vi "main.vi"() -> ()   [LabVIEW 2016]
uses:
  global/Config_Infos.vi
  <vilib>/registry/registry.llb/Registry RtKey.ctl
  <vilib>/registry/registry.llb/Read Registry Value Simple STR.vi
panel:
  out "String/Binary data":string
  in  "config file":path=path "C:/Users/guigue/Documents/hardware/software_config/rga/RGAConfig.ini"
  in  "stop":bool
  in  "Tab Control":enum32{"Status", "Ping listener", "Log"}(tab)
  in  "saving?":bool
  in  "filament?":bool
  out "status display":u16(ring)=5 items=["Filament on/Saving off", "Waiting 1", "Filament on/Saving on", "Waiting 2", "Filament off/Saving off", "Idle"]
  out "Init OK?":bool
  out "error initialization (out)":errorcluster
  out "broadcast.ping listener?":bool=TRUE
  in  "is_running?":bool
  in  "is_stopping?":bool
  out "broadcast.ping error out":errorcluster
  out "Execution:State":T1(ring)
  out "service log":string
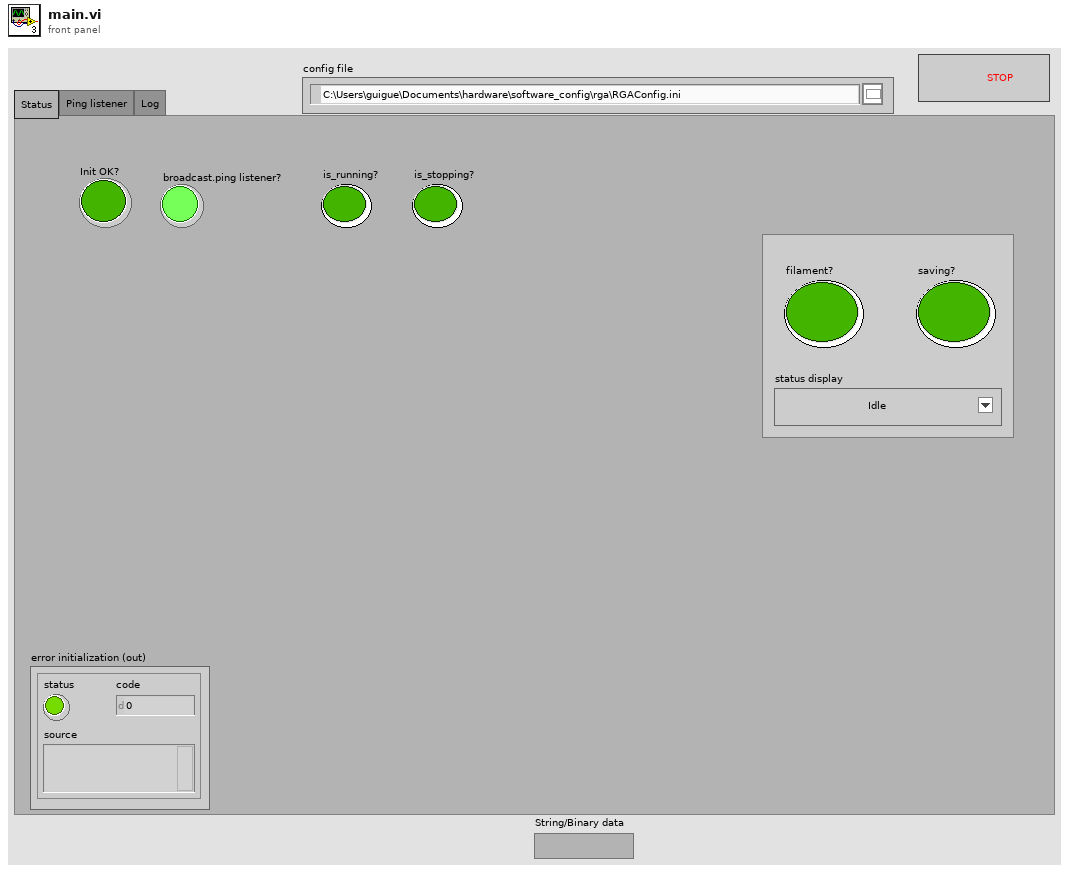
[diagram p1: front panel]
types:
  T1 = enum32{"Bad", "Idle", "Run top level", "Running"}
  T2 = typedef "Registry RtKey.ctl" = enum32{"HKEY_CLASSES_ROOT", "HKEY_CURRENT_USER", "HKEY_LOCAL_MACHINE", "HKEY_USERS", "HKEY_PERFORMANCE_DATA", "HKEY_CURRENT_CONFIG", "HKEY_DYN_DATA"}
  T3 = typedef "Registry refnum.ctl" = refnum<k1>
  T4 = cluster{"stop":refnum<vi>, "is_running?":refnum<vi>, "is_stopping?":refnum<vi>, "filament?":refnum<vi>, "saving?":refnum<vi>, "status display":refnum<vi>}
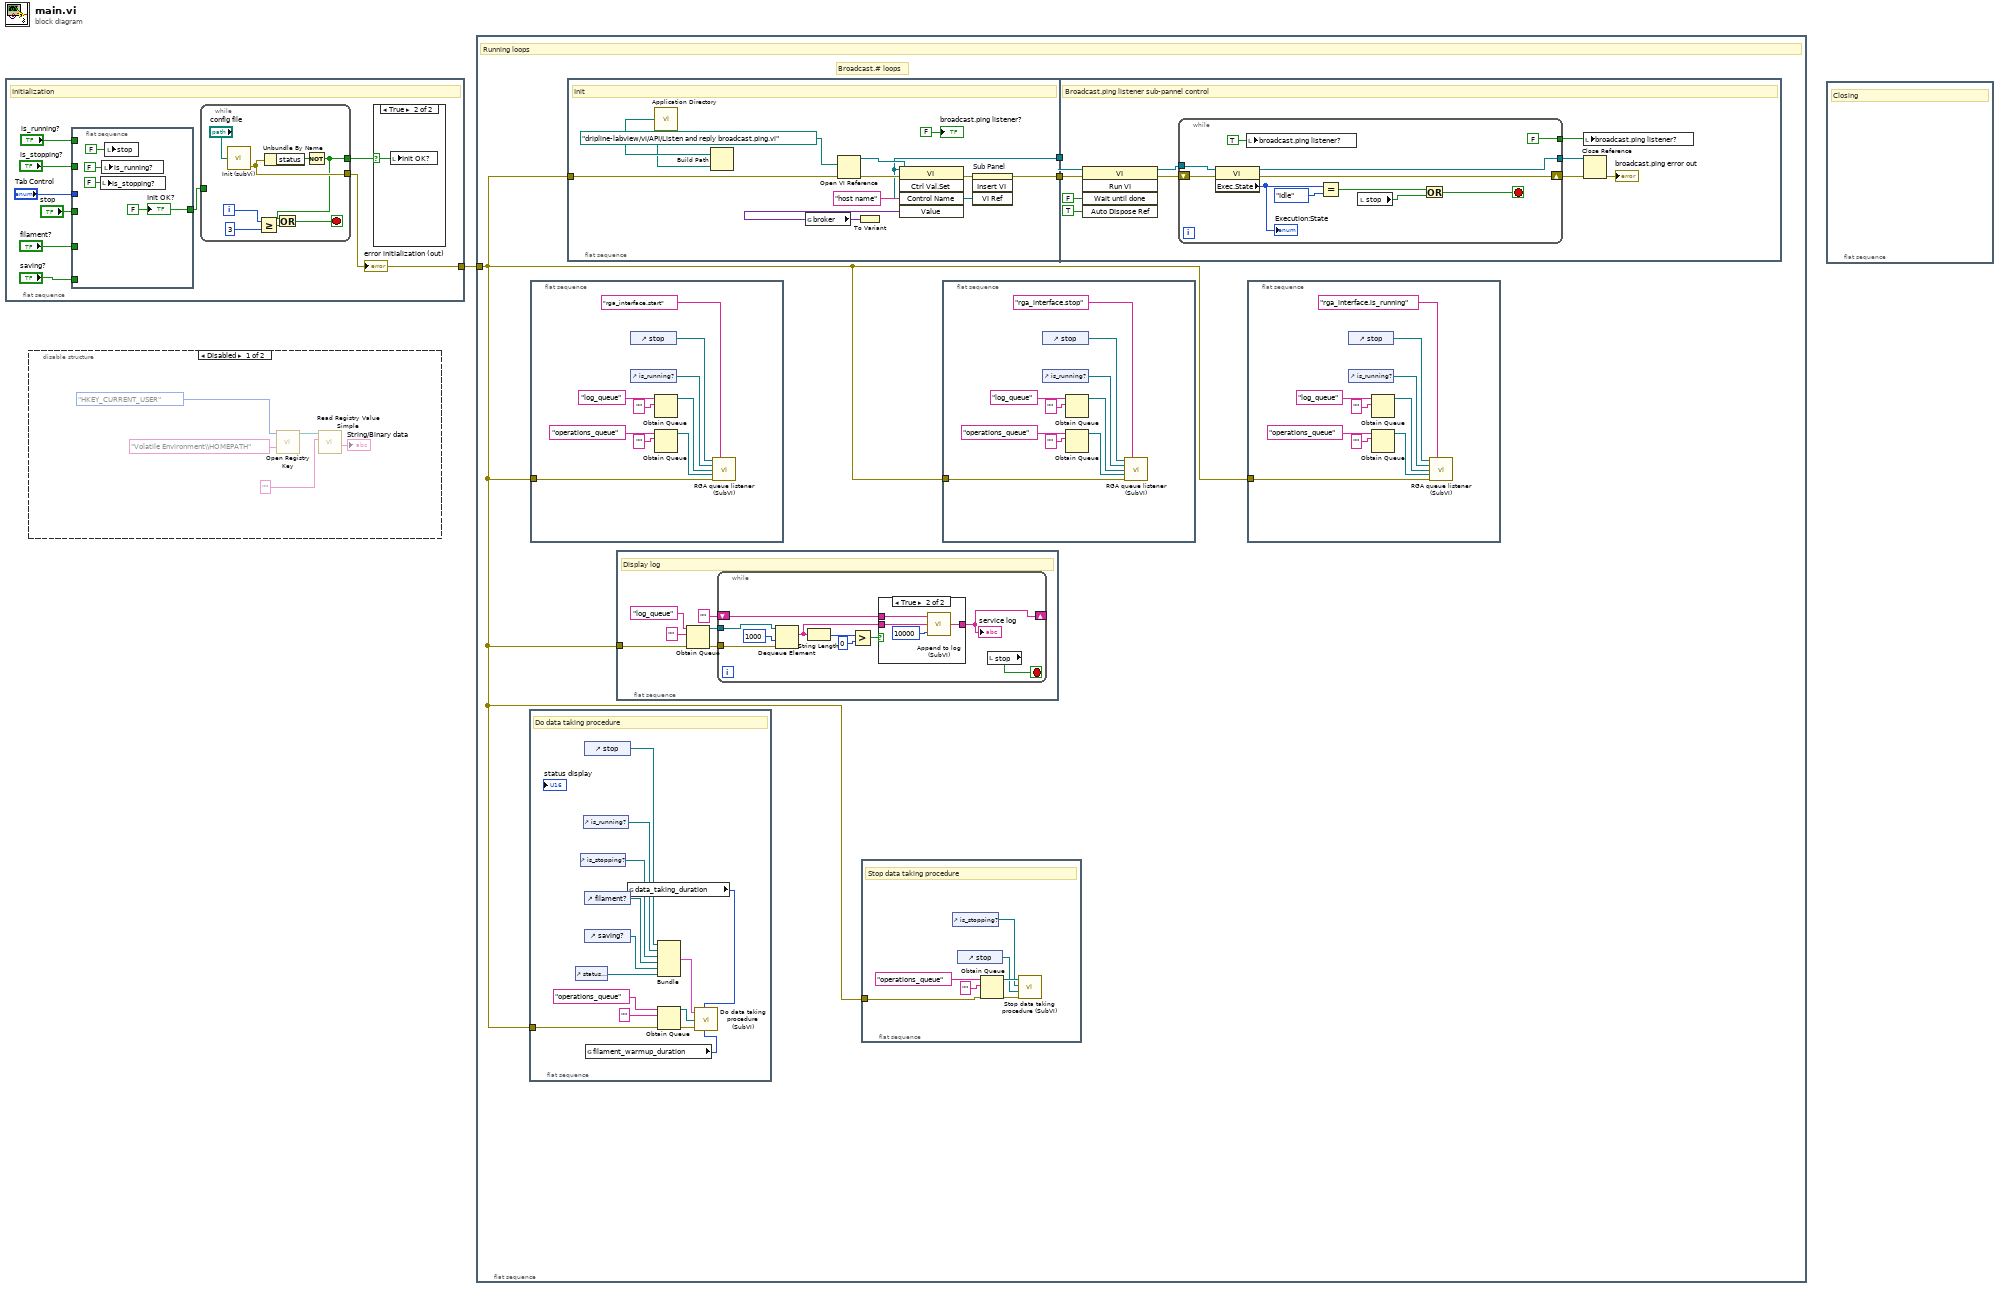
[diagram p0: block diagram]
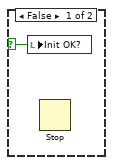
[diagram p4: hidden frame]
diagram:
  n1 = flat-sequence {
    tunnel: [w8] -> w1
    frame #0 {
      # "Initialization"
      n2 = flat-sequence {
        tunnel: [w14] -> w9
        tunnel: "stop" -> [_]
        tunnel: "Tab Control" -> [_]
        tunnel: "is_running?" -> [_]
        tunnel: "is_stopping?" -> [_]
        tunnel: "filament?" -> [_]
        tunnel: "saving?" -> [_]
        frame #0 {
          w14 = FALSE ("Init OK?")
          n3 = local write "is_stopping?"(FALSE ("stop")) -> ()
          n4 = local write "is_running?"(FALSE ("stop")) -> ()
          n5 = local write "stop"(FALSE ("stop")) -> ()
          "Init OK?" <- w14
        }
      }
      n6 = while {
        tunnel: [w18] -> w10
        tunnel: [w19] -> w8
        tunnel: w9 -> [_]
        i -> [w22]
        stop <- w24 stop-if-true
        n7 = call "Init (subVi).vi"("config file"="config file") -> ("error (out)"=w19:errorcluster)  [unwired: 2 in]
        n8 = Greater Or Equal?(x=w22, y=3) -> (x >= y?=w23:bool)
        n9 = Unbundle By Name(w19) -> ("status"=w20:bool)
        n10 = Not(x=w20) -> (.not. x?=w18:bool)
        n11 = Or(x=w18, y=w23) -> (x .or. y?=w24:bool)
      }
      "error initialization (out)" <- w8
      n12 = case shown="True" w10 {
        selector: w10 -> [w15 w16]
        frame False {
          n13 = local write "Init OK?"(w15) -> ()
          n14 = Stop() -> ()  [unwired: 1 in]
        }
        frame True {
          n15 = local write "Init OK?"(w16) -> ()
        }
      }
    }
  }
  n16 = disable-structure shown="Disabled" {
    frame Disabled {
      n17 = call <vilib>:"Open Registry Key.vi"("subkey"="Volatile Environment\\HOMEPATH", "root key (HKEY_LOCAL_MACHINE)"=Registry_RtKey."HKEY_CURRENT_USER") -> ("refnum out"=w27:T3)  [unwired: 8 in, 1 out]
      n18 = call-poly <vilib>:"Read Registry Value Simple.vi"("value"="", "refnum"=w27) -> ("String/Binary data"=→"String/Binary data":string)  [unwired: 4 in, 3 out]
    }
    frame Enabled {
    }
  }
  n19 = flat-sequence {
    tunnel: w1 -> [w30]
    frame #0 {
      # "Broadcast.# loops"
      # "Running loops"
      n20 = flat-sequence {
        tunnel: w30 -> [w91]
        frame #0 {
          # "Do data taking procedure"
          n21 = control-ref of="status display"() -> (w85:refnum<vi>)
          n22 = control-ref of="is_stopping?"() -> (w87:refnum<vi>)
          n23 = control-ref of="is_running?"() -> (w88:refnum<vi>)
          n24 = control-ref of="stop"() -> (w89:refnum<vi>)
          n25 = control-ref of="filament?"() -> (w86:refnum<vi>)
          n26 = control-ref of="saving?"() -> (w84:refnum<vi>)
          n27 = global read "Config_Infos.vi" "filament_warmup_duration"() -> (w81:i32)
          n28 = global read "Config_Infos.vi" "data_taking_duration"() -> (w82:i32)
          n29 = Bundle("stop"=w89, "is_running?"=w88, "is_stopping?"=w87, "filament?"=w86, "saving?"=w84, "status display"=w85) -> (w83:T4)  [unwired: 1 in]
          n30 = Obtain Queue(name (unnamed)="operations_queue", element data type="", error in (no error)=w91) -> (queue out=w92:refnum<queue>, error out=w90:errorcluster)  [unwired: 2 in, 1 out]
          n31 = call "Do data taking procedure (SubVI).vi"("input cluster"=w83, "duration data taking (s)"=w82, "queue in"=w92, "error in (no error)"=w90, "filament warmup duration (s)"=w81) -> ()  [unwired: 1 in, 1 out]
        }
      }
      n32 = flat-sequence {
        tunnel: w30 -> [w104]
        frame #0 {
          n33 = control-ref of="stop"() -> (w96:refnum<vi>)
          n34 = control-ref of="is_running?"() -> (w95:refnum<vi>)
          n35 = Obtain Queue(name (unnamed)="log_queue", element data type="") -> (queue out=w97:refnum<queue>)  [unwired: 3 in, 2 out]
          n36 = Obtain Queue(name (unnamed)="operations_queue", element data type="") -> (queue out=w102:refnum<queue>)  [unwired: 3 in, 2 out]
          n37 = call "RGA queue listener (SubVI).vi"("stop bool"=w96, "binding key"="rga_interface.start", "is_running bool"=w95, "log queue in"=w97, "queue in"=w102, "error in (no error)"=w104) -> ()  [unwired: 9 in, 1 out]
        }
      }
      n38 = flat-sequence {
        tunnel: [w108] -> w32
        tunnel: [w109] -> w31
        tunnel: w30 -> [w107]
        tunnel: w32 -> [w120]
        tunnel: w31 -> [w119]
        frame #0 {
          w105 = path "dripline-labview/vi/API/Listen and reply broadcast.ping.vi" ("vi path")
          # "Init"
          n39 = call <vilib>:"Application Directory.vi"() -> ("Application Directory"=w106:path)
          n40 = Build Path(base path=w106, name or relative path=w105) -> ()  [unwired: 1 out]
          n41 = global read "Config_Infos.vi" "broker"() -> (w113:string)
          n42 = Open VI Reference(vi path=w105, error in (no error)=w107) -> (vi reference=w111:refnum<vi>, error out=w114:errorcluster)  [unwired: 4 in]
          n43 = To Variant(anything=w113) -> (Variant=w115:variant)
          n44 = invoke class="VI" method="Ctrl Val.Set"(reference=w111, error in=w114, "Control Name"="host name", "Value"=w115) -> (reference out=w108:refnum<vi>, error out=w110:errorcluster)  [unwired: 1 in, 3 out]
          n45 = invoke on="Sub Panel" class="SubPnl" method="Insert VI"(error in=w110, "VI Ref"=w108) -> (error out=w109:errorcluster)  [unwired: 2 in, 3 out]
          "broadcast.ping listener?" <- FALSE ("Boolean")
        }
        frame #1 {
          # "Broadcast.ping listener sub-pannel control"
          n46 = invoke class="VI" method="Run VI"(reference=w120, error in=w119, "Wait until done"=FALSE ("Wait Until Done"), "Auto Dispose Ref"=TRUE ("Auto Dispose Reference")) -> (reference out=w125:refnum<vi>, error out=w118:errorcluster)  [unwired: 1 in, 3 out]
          n47 = while {
            tunnel: w125 -> [w135]
            tunnel: [w134] -> w124
            tunnel: [FALSE] -> w121
            shift-right: [w127] -> w117
            shift-left: w118 -> [w128]
            stop <- w130 stop-if-true
            n48 = property class="VI"(reference=w135, error in=w128) -> (reference out=w134:refnum<vi>, error out=w127:errorcluster, "Exec.State"=w132:T1)
            "Execution:State" <- w132
            n49 = local write "broadcast.ping listener?"(TRUE ("broadcast.ping listener?")) -> ()
            n50 = Equal?(x=w132, y=T1."Idle") -> (x = y?=w129:bool)
            n51 = local read "stop"() -> (w133:bool)
            n52 = Or(x=w129, y=w133) -> (x .or. y?=w130:bool)
          }
          n53 = local write "broadcast.ping listener?"(w121) -> ()
          n54 = Close Reference(reference=w124, error in (no error)=w117) -> (error out=→"broadcast.ping error out":errorcluster)
        }
      }
      n55 = flat-sequence {
        tunnel: w30 -> [w63]
        frame #0 {
          # "Display log"
          n56 = Obtain Queue(name (unnamed)="log_queue", element data type="", error in (no error)=w63) -> (queue out=w62:refnum<queue>, error out=w61:errorcluster)  [unwired: 2 in, 1 out]
          n57 = while {
            tunnel: w62 -> [w75]
            tunnel: w61 -> [w73]
            shift-right: [w71] -> _
            shift-left: "" ("log out") -> [w72]
            stop <- w74 stop-if-true
            n58 = Dequeue Element(queue=w75, timeout in ms (-1)=1000, error in (no error)=w73) -> (element=w66:string)  [unwired: 3 out]
            n59 = String Length(string=w66) -> (length=w69:i32)
            n60 = Greater?(x=w69, y=0) -> (0:w67:bool)
            n61 = case shown="True" w67 {
              tunnel: w72 -> [w76 w80]
              tunnel: [w76 w79] -> w71
              tunnel: w66 -> [_ w77]
              frame False {
              }
              frame True {
                n62 = call "Append to log (SubVI).vi"("log length"=10000, "to append"=w77, "log in"=w80) -> ("log out"=w79:string)
              }
            }
            "service log" <- w71
            n63 = local read "stop"() -> (w74:bool)
          }
        }
      }
      n64 = flat-sequence {
        tunnel: w30 -> [w33]
        frame #0 {
          # "Stop data taking procedure"
          n65 = control-ref of="is_stopping?"() -> (w34:refnum<vi>)
          n66 = control-ref of="stop"() -> (w35:refnum<vi>)
          n67 = Obtain Queue(name (unnamed)="operations_queue", element data type="", error in (no error)=w33) -> (queue out=w37:refnum<queue>, error out=w36:errorcluster)  [unwired: 2 in, 1 out]
          n68 = call "Stop data taking procedure (SubVI).vi"("error in (no error)"=w36, "stop"=w35, "is_stopping?"=w34, "Queue in"=w37) -> ()  [unwired: 1 in, 1 out]
        }
      }
      n69 = flat-sequence {
        tunnel: w30 -> [w59]
        frame #0 {
          n70 = control-ref of="stop"() -> (w51:refnum<vi>)
          n71 = control-ref of="is_running?"() -> (w50:refnum<vi>)
          n72 = Obtain Queue(name (unnamed)="log_queue", element data type="") -> (queue out=w52:refnum<queue>)  [unwired: 3 in, 2 out]
          n73 = Obtain Queue(name (unnamed)="operations_queue", element data type="") -> (queue out=w57:refnum<queue>)  [unwired: 3 in, 2 out]
          n74 = call "RGA queue listener (SubVI).vi"("stop bool"=w51, "binding key"="rga_interface.stop", "is_running bool"=w50, "log queue in"=w52, "queue in"=w57, "error in (no error)"=w59) -> ()  [unwired: 9 in, 1 out]
        }
      }
      n75 = flat-sequence {
        tunnel: w30 -> [w49]
        frame #0 {
          n76 = control-ref of="stop"() -> (w41:refnum<vi>)
          n77 = control-ref of="is_running?"() -> (w40:refnum<vi>)
          n78 = Obtain Queue(name (unnamed)="log_queue", element data type="") -> (queue out=w42:refnum<queue>)  [unwired: 3 in, 2 out]
          n79 = Obtain Queue(name (unnamed)="operations_queue", element data type="") -> (queue out=w47:refnum<queue>)  [unwired: 3 in, 2 out]
          n80 = call "RGA queue listener (SubVI).vi"("stop bool"=w41, "binding key"="rga_interface.is_running", "is_running bool"=w40, "log queue in"=w42, "queue in"=w47, "error in (no error)"=w49) -> ()  [unwired: 9 in, 1 out]
        }
      }
    }
  }
  n81 = flat-sequence {
    frame #0 {
      # "Closing"
    }
  }
